vi "Set Level Offset.vi"(8 "error in (no error)":errorcluster, 9 "Level Offset (0) [V]":dbl, 10 "Output BNC (T0)":T1 items=["T0", "AB", "CD", "EF", "GH"], 11 "VISA resource name":refnum<visa-resource-name>) -> (0 "error out":errorcluster, 3 "VISA resource name out":refnum<visa-resource-name>, 4 "Device Errors":cluster{"code":i32, "Text":string}[](array[cluster]))   [LabVIEW 2014, in "Stanford Research DG645 - Driver.lvlib"]
doc: "Delay and Output Command: LOFF b,v\nInstrument Error Check\n\nSet the level offset for output b to v (in volt)."
uses:
  Stanford Research DG645 - Driver.lvlib
  Output BNC.ctl
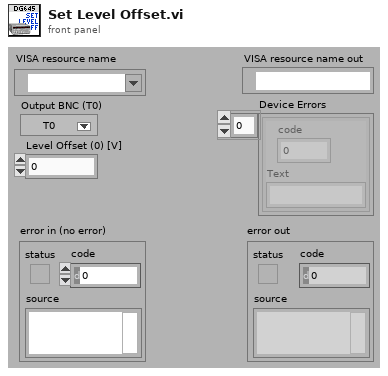
[diagram p1: front panel]
types:
  T1 = typedef "Stanford Research DG645 - Driver.lvlib/Output BNC.ctl" = i32
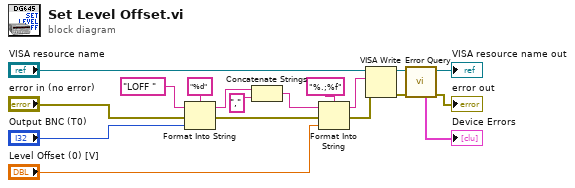
[diagram p0: block diagram]
diagram:
  n1 = Format Into String(format string="%d", initial string="LOFF " ("command"), error in="error in (no error)", "Output BNC (T0)") -> (resulting string=w2:string, error out=w1:errorcluster)
  n2 = Concatenate Strings(w2, "," ("command")) -> (w11:string)
  n3 = Format Into String(format string="%.;%f", initial string=w11, error in=w1, "Level Offset (0) [V]") -> (resulting string=w13:string, error out=w8:errorcluster)
  n4 = VISA Write(VISA resource name="VISA resource name", write buffer=w13, error in (no error)=w8) -> (VISA resource name out=w9:refnum<visa-resource-name>, error out=w5:errorcluster)  [unwired: 1 out]
  n5 = call "Error Query.vi"("error in (no error)"=w5, "VISA resource name"=w9) -> ("error out"=→"error out":errorcluster, "VISA resource name out"=→"VISA resource name out":refnum<visa-resource-name>, "Device Errors"=→"Device Errors":cluster{"code":i32, "Text":string}[])  [unwired: 7 in]
